vi "Update Status.vi"(7 "Check overlay?":bool, 8 "error in (no error)":errorcluster, 9 "Status":T1=enum."Passed", 10 "Case":string, 11 "Icon Decorator In":refnum<class "Icon Decorator.lvclass">) -> (0 "error out":errorcluster)   [LabVIEW 2020, in "Icon Decorator.lvlib" / "Icon Decorator.lvclass"]
uses:
  Icon Decorator.lvclass
  Core/Result/Status.ctl
  Core/Result/Result.lvlib
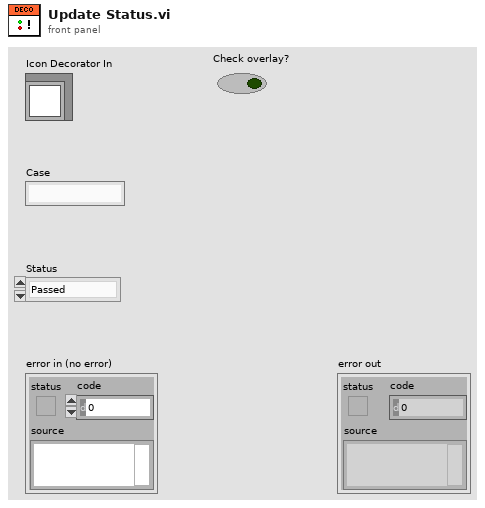
[diagram p1: front panel]
types:
  T1 = typedef "Result.lvlib/Status.ctl" = enum16{"", "Passed", "Failed", "Error", "Skipped", "Setup Error", "Broken", "Teardown Error"}
  T2 = typedef "ItemRef.ctl" = u64
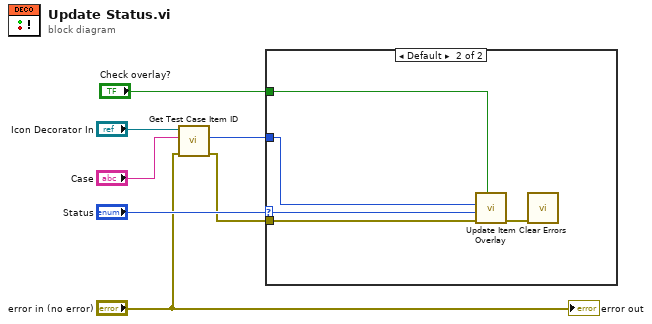
[diagram p0: block diagram]
diagram:
  n1 = call "Get Test Case Item ID.vi"("error in (no error)"="error in (no error)", "Test Case"="Case", "Icon Decorator In"="Icon Decorator In") -> ("error out"=w3:errorcluster, "ObjectItem"=w4:T2)  [unwired: 7 in]
  n2 = case shown="Default" "Status" {
    selector: "Status" -> [_ w9]
    tunnel: w4 -> [_ w12]
    tunnel: w3 -> [_ w11]
    tunnel: "Check overlay?" -> [_ w8]
    frame "" {
    }
    frame Default {
      n3 = call "Update Item Overlay.vi"("Check overlay?"=w8, "error in (no error)"=w11, "Status"=w9, "Item"=w12) -> ("error out"=w10:errorcluster)  [unwired: 7 in]
      n4 = call <vilib>:"Clear Errors.vi"("error in (no error)"=w10) -> ()  [unwired: 5 in, 2 out]
    }
  }
  "error out" <- "error in (no error)"
